vi "getRx.vi"(6 "Vx":dbl, 8 "理论 K":dbl, 9 "R5-1":dbl, 10 "传感器索引":i32, 11 "数据":dbl[][](array[numeric])) -> (3 "Rx":dbl)   [LabVIEW 2017]
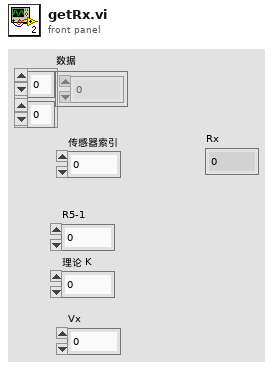
[diagram p1: front panel]
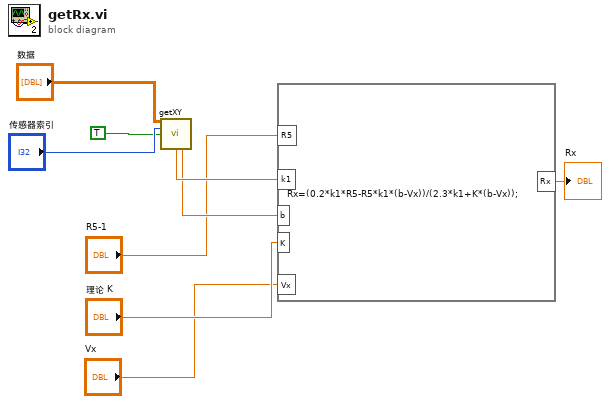
[diagram p0: block diagram]
diagram:
  n1 = call "getXY.vi"("数据"="数据", "传感器索引"="传感器索引", "是否需要计算拟合曲线"=TRUE) -> ("slope"=w6:dbl, "intercept"=w5:dbl)  [unwired: 5 in, 6 out]
  n2 = formula code="Rx=(0.2*k1*R5-R5*k1*(b-Vx))/(2.3*k1+K*(b-Vx));"("k1"=w6, "R5"="R5-1", "K"="理论 K", "b"=w5, "Vx"="Vx") -> ("Rx"=→"Rx":dbl)
